vi "Open_SRP_Socket.vi"(8 "error in (no error)":errorcluster, 9 "Bypass Ducat AutoSearch":bool, 10 "Ducat Name":string="ducat3", 11 "SRP Server Name":string="jit3") -> (0 "error out":errorcluster, 2 "Data Out":string, 3 "TCP Network Connection out":refnum<k5>)   [LabVIEW 2011]
doc: "This VI opens the socket to the SRP for communication for a specified ducat and server..\n\nInputs:\n1. SRP Server Name: (jit1, jit2, jit3, jitterbug)\n2. Ducat Name: Ducat your workstation is attached to (ducat1, ducat2, ducat3, etc.)\n3. Bypass Ducat AutoSearch: If False (off), the ducat will be automatically selected by pinging each ducat according to the testers.txt file. If True (on), the Ducat Name field will be utilized.\n\nOutputs:\n1. Data Out: SRP System Response read from Socket\n2. TCP Network Connection Out: Specified socket number."
uses:
  <vilib>/Utility/error.llb/DialogType.ctl
  Global_SRP_Socket.vi
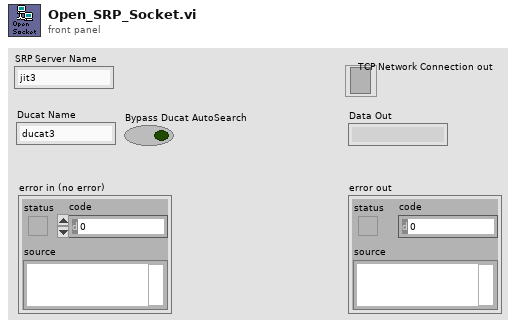
[diagram p1: front panel]
types:
  T1 = typedef "DialogType.ctl" = u16
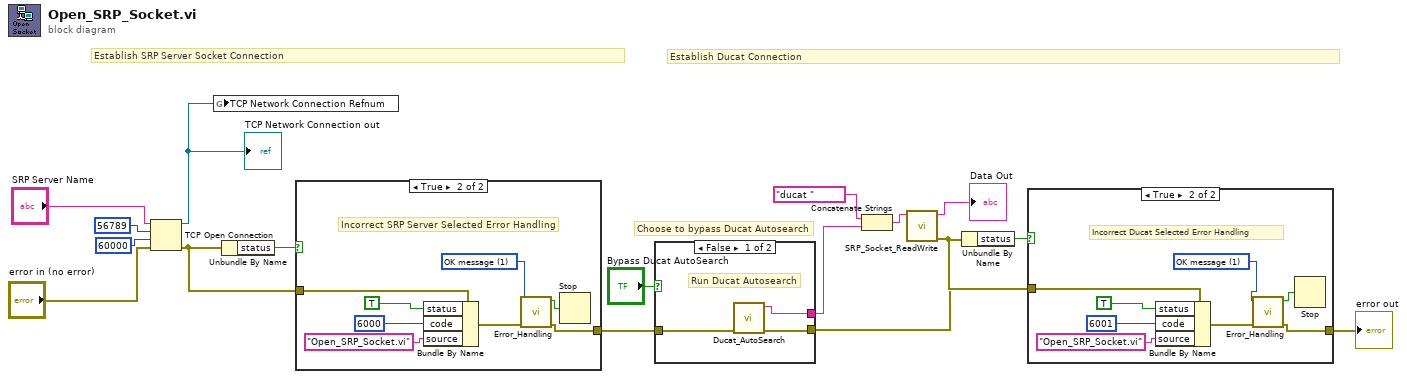
[diagram p0: block diagram]
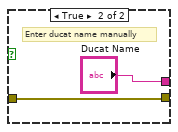
[diagram p2: hidden frame]
diagram:
  # "Choose to bypass Ducat Autosearch"
  # "Establish Ducat Connection"
  # "Establish SRP Server Socket Connection"
  n1 = TCP Open Connection(address="SRP Server Name", remote port or service name=u16 56789, timeout ms (60000)=60000, error in (no error)="error in (no error)") -> (connection ID=w12:refnum<k5>, error out=w11:errorcluster)  [unwired: 1 in]
  "TCP Network Connection out" <- w12
  n2 = global write "Global_SRP_Socket.vi" "TCP Network Connection Refnum"(w12) -> ()
  n3 = Unbundle By Name(w11) -> ("status"=w10:bool)
  n4 = case shown="True" w10 {
    tunnel: w11 -> [w18 w23]
    tunnel: [w18 w21] -> w5
    frame False {
    }
    frame True {
      w20 = T1 1 items=["no dialog", "OK message", "continue or stop message", "OK message + warnings", "continue/stop + warnings"] ("type of dialog (OK msg:1)")
      # "Incorrect SRP Server Selected Error Handling"
      n5 = Bundle By Name(cluster=w23, "status"=TRUE, "code"=6000, "source"="Open_SRP_Socket.vi") -> (w22:errorcluster)
      n6 = call "Error_Handling.vi"("error in (no error)"=w22, "type of dialog (OK msg:1)"=w20) -> ("error out"=w21:errorcluster, "error?"=w19:bool)  [unwired: 8 in]
      n7 = Stop(stop? (T)=w19) -> ()
    }
  }
  n8 = case shown="False" "Bypass Ducat AutoSearch" {
    tunnel: [w29 w30] -> w6
    tunnel: w5 -> [w28 w30]
    tunnel: [w27 "Ducat Name"] -> w3
    frame False {
      # "Run Ducat Autosearch"
      n9 = call "Ducat_AutoSearch.vi"("error in"=w28) -> ("error out"=w29:errorcluster, "Ducat Number"=w27:string)  [unwired: 9 in]
    }
    frame True {
      # "Enter ducat name manually"
    }
  }
  n10 = Concatenate Strings("ducat ", w3) -> (w2:string)
  n11 = call "SRP_Socket_ReadWrite.vi"("error in (no error)"=w6, "Data In"=w2) -> ("error out"=w7:errorcluster, "Data Out"=→"Data Out":string)  [unwired: 7 in]
  n12 = Unbundle By Name(w7) -> ("status"=w8:bool)
  n13 = case shown="True" w8 {
    tunnel: w7 -> [w32 w37]
    tunnel: [w32 w35] -> w16
    frame False {
    }
    frame True {
      w34 = T1 1 items=["no dialog", "OK message", "continue or stop message", "OK message + warnings", "continue/stop + warnings"] ("type of dialog (OK msg:1)")
      # "Incorrect Ducat Selected Error Handling"
      n14 = Bundle By Name(cluster=w37, "status"=TRUE, "code"=6001, "source"="Open_SRP_Socket.vi") -> (w36:errorcluster)
      n15 = call "Error_Handling.vi"("error in (no error)"=w36, "type of dialog (OK msg:1)"=w34) -> ("error out"=w35:errorcluster, "error?"=w33:bool)  [unwired: 8 in]
      n16 = Stop(stop? (T)=w33) -> ()
    }
  }
  "error out" <- w16
